vi "UpdateDataExplorerSpecificFeatureListProperty.vi"(5 "features":string[](array[string]), 7 "display names":string[](array[string]), 8 "error in (no error)":errorcluster, 9 "channel":string, 10 "group":string="Waveforms", 11 "TDMS ref in":refnum<k34>) -> (0 "error out":errorcluster, 1 "channel name out":string, 2 "group name out":string, 3 "TDMS ref out":refnum<k34>)   [LabVIEW 2017, in "Tdms.lvlib"]
uses:
  <vilib>/addons/InsightCM/Utilities/Tdms/Tdms.lvlib
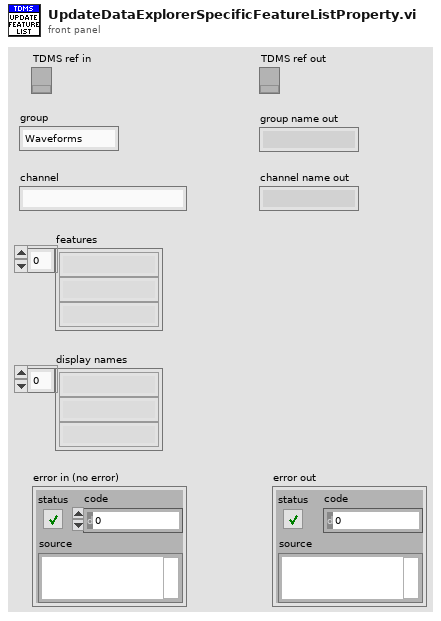
[diagram p1: front panel]
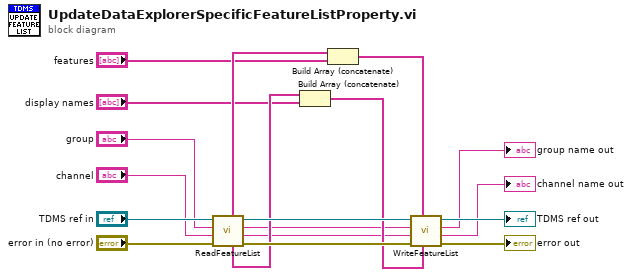
[diagram p0: block diagram]
diagram:
  n1 = call <vilib>:"ReadFeatureList.vi"("error in (no error)"="error in (no error)", "Channel"="channel", "Group"="group", "TDMS Ref In"="TDMS ref in") -> ("error out"=w14:errorcluster, "Channel Name Out"=w5:string, "Group Name Out"=w6:string, "TDMS Ref Out"=w13:refnum<k34>, "Feature Display Names"=w9:string[], "Feature Code Names"=w12:string[])  [unwired: 2 in]
  n2 = Build Array (concatenate)(w9, "display names") -> (w7:string[])
  n3 = Build Array (concatenate)(w12, "features") -> (w10:string[])
  n4 = call <vilib>:"WriteFeatureList.vi"("Feature Display Names"=w7, "Feature Code Names"=w10, "error in (no error)"=w14, "Channel Name In"=w5, "Group Name In"=w6, "TDMS Ref In"=w13) -> ("error out"=→"error out":errorcluster, "Channel Name Out"=→"channel name out":string, "Group Name Out"=→"group name out":string, "TDMS Ref Out"=→"TDMS ref out":refnum<k34>)  [unwired: 2 in]
